vi "kinematics.vi"(11 "input":dbl[](array[numeric])) -> (1 "result":dbl[][](array[numeric]), 2 "position":dbl[](array[numeric]), 3 "length":dbl[](array[numeric]))   [LabVIEW 2018]
uses:
  <vilib>/Analysis/_algsub.llb/Real Vector Norm.vi
  <vilib>/Analysis/Matrix/Numeric/Conversions/Array To Matrix - RA2.vi
  <vilib>/Analysis/Matrix/Numeric/Multiply/Multiply - RM,RM.vi
  <vilib>/Analysis/Matrix/Numeric/Subtract/Subtract - RM,RM.vi
  <vilib>/Analysis/Matrix/Numeric/Add/Add - RM,RM.vi
  <vilib>/Analysis/Matrix/Numeric/Conversions/Matrix To Array - RM.vi
  <vilib>/Analysis/NI_AALPro.lvlib
  <vilib>/Analysis/Matrix/NI_Matrix.lvlib
panel:
  # "(X, Y, Z)"
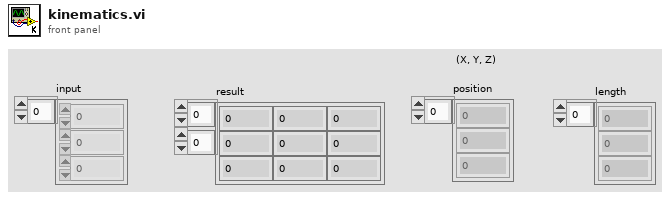
[diagram p1: front panel]
types:
  T1 = typedef "NI_Matrix.lvlib/RealMatrix.ctl" = dbl[][]
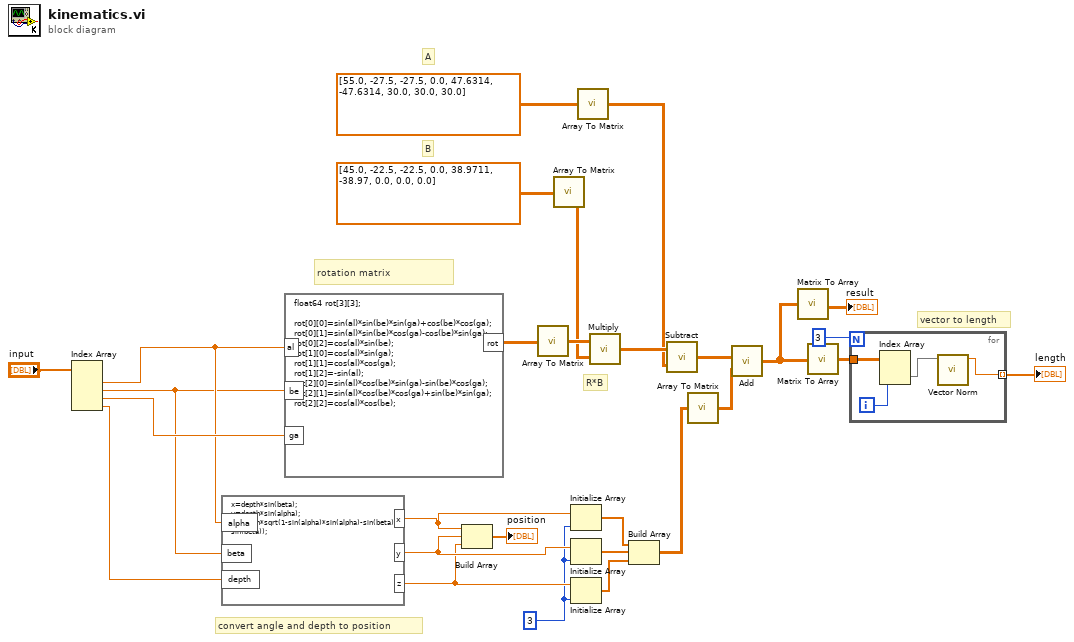
[diagram p0: block diagram]
diagram:
  w8 = 3
  # "convert angle and depth to position"
  # "A"
  # "B"
  # "rotation matrix"
  # "vector to length"
  # "R*B"
  n1 = Index Array(array="input") -> (element #1=w3:dbl, element #2=w2:dbl, element #3=w4:dbl, element #4=w1:dbl)  [unwired: 4 in]
  n2 = formula code="x=depth*sin(beta);\ny=depth*sin(alpha);\nz=depth*sqrt(1-sin(alpha)*sin(alpha)-sin(beta)*sin(beta));"("alpha"=w3, "beta"=w2, "depth"=w1) -> ("x"=w11:dbl, "y"=w10:dbl, "z"=w9:dbl)
  n3 = formula code="float64 rot[3][3];\n\nrot[0][0]=sin(al)*sin(be)*sin(ga)+cos(be)*cos(ga);\nrot[0][1]=sin(al)*sin(be)*cos(ga)-cos(be)*sin(ga);\nrot[0][2]=cos(al)*sin(be);\nrot[1][0]=cos(al)*sin(ga);\nrot[1][1]=cos(al)*cos(ga);\nrot[1][2]=-sin(al);\nrot[2][0]=sin(al)*cos(be)*sin(ga)-sin(be)*cos(ga);\nrot[2][1]=sin(al)*cos(be)*cos(ga)+sin(be)*sin(ga);\nrot[2][2]=cos(al)*cos(be);"("al"=w3, "be"=w2, "ga"=w4) -> ("rot"=w18:dbl[][])
  n4 = Build Array(w11, w10, w9) -> (→"position":dbl[])
  n5 = call-poly <vilib>:"Array To Matrix.vi"("Real 2D Array"=w18) -> ("Real Matrix"=w25:T1)
  n6 = call-poly <vilib>:"Array To Matrix.vi"("Real 2D Array"=dbl[][] [[45.0, -22.5, -22.5], [0.0, 38.9711, -38.97], [0.0, 0.0, 0.0]]) -> ("Real Matrix"=w24:T1)
  n7 = Initialize Array(w11, w8) -> (w12:dbl[])
  n8 = Initialize Array(w10, w8) -> (w13:dbl[])
  n9 = Initialize Array(w9, w8) -> (w14:dbl[])
  n10 = call-poly <vilib>:"Array To Matrix.vi"("Real 2D Array"=dbl[][] [[55.0, -27.5, -27.5], [0.0, 47.6314, -47.6314], [30.0, 30.0, 30.0]]) -> ("Real Matrix"=w22:T1)
  n11 = call-poly <vilib>:"Multiply.vi"("Real Matrix B"=w24, "Real Matrix A"=w25) -> ("A * B"=w28:T1)
  n12 = Build Array(w12, w13, w14) -> (w7:dbl[][])
  n13 = call-poly <vilib>:"Subtract.vi"("Real Matrix B"=w22, "Real Matrix A"=w28) -> ("A - B"=w26:T1)
  n14 = call-poly <vilib>:"Array To Matrix.vi"("Real 2D Array"=w7) -> ("Real Matrix"=w23:T1)
  n15 = call-poly <vilib>:"Add.vi"("Real Matrix B"=w23, "Real Matrix A"=w26) -> ("A + B"=w20:T1)
  n16 = call-poly <vilib>:"Matrix To Array.vi"("Real Matrix"=w20) -> ("Real 2D Array"=→"result":dbl[][])
  n17 = call-poly <vilib>:"Matrix To Array.vi"("Real Matrix"=w20) -> ("Real 2D Array"=w19:dbl[][])
  n18 = for {
    N: 3 -> [_]
    tunnel: w19 -> [w32]
    tunnel: [w30] -> w6 mode=indexing
    i -> [w31]
    n19 = Index Array(array=w32, index (col)=w31) -> (element=w29:dbl[])  [unwired: 1 in]
    n20 = call-poly <vilib>:"Vector Norm.vi"("Input Vector"=w29) -> ("norm"=w30:dbl)  [unwired: 9 in, 1 out]
  }
  "length" <- w6
